vi "Set Button Positions.vi"(4 "Left":i16, 6 "Top":i32, 8 "error in":errorcluster, 10 "label array in":string[](array[string]), 11 "controls[] in":refnum<vi>[](array[refnum])) -> (0 "error out":errorcluster)   [LabVIEW 2018]
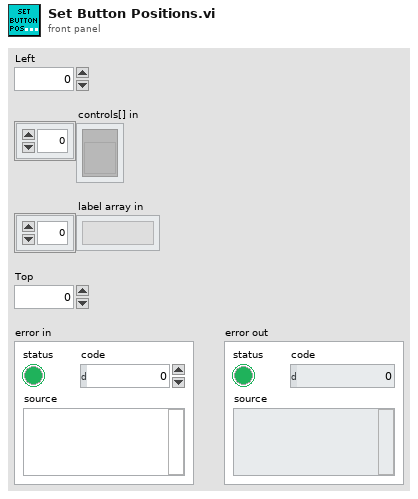
[diagram p1: front panel]
types:
  T1 = typedef "LVRectTypeDef.ctl" = cluster{"Left":i16, "Top":i16, "Right":i16, "Bottom":i16}
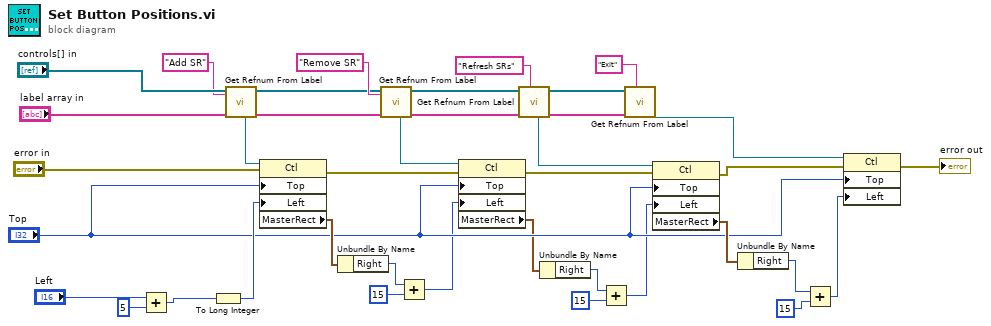
[diagram p0: block diagram]
diagram:
  n1 = Add(x="Left", y=i16 5) -> (x+y=w2:i16)
  n2 = To Long Integer(number=w2) -> (32bit integer=w20:i32)
  n3 = call "Get Refnum From Label.vi"("label"="Add SR" ("element"), "label array in"="label array in", "controls[] in"="controls[] in") -> ("label array out"=w16:string[], "controls[] out"=w17:refnum<vi>[], "refnum out"=w32:refnum<vi>)  [unwired: 6 in]
  n4 = property class="Ctl"(reference=w32, error in="error in", "Top"="Top", "Left"=w20) -> (error out=w13:errorcluster, "MasterRect"=w28:T1)  [unwired: 1 out]
  n5 = Unbundle By Name(w28) -> ("Right"=w29:i16)
  n6 = call "Get Refnum From Label.vi"("label"="Remove SR" ("element"), "label array in"=w16, "controls[] in"=w17) -> ("label array out"=w15:string[], "controls[] out"=w14:refnum<vi>[], "refnum out"=w4:refnum<vi>)  [unwired: 6 in]
  n7 = Add(x=w29, y=i16 15) -> (x+y=w9:i16)
  n8 = property class="Ctl"(reference=w4, error in=w13, "Top"="Top", "Left"=w9) -> (error out=w11:errorcluster, "MasterRect"=w6:T1)  [unwired: 1 out]
  n9 = call "Get Refnum From Label.vi"("label"="Refresh SRs" ("element"), "label array in"=w15, "controls[] in"=w14) -> ("label array out"=w36:string[], "controls[] out"=w37:refnum<vi>[], "refnum out"=w35:refnum<vi>)  [unwired: 6 in]
  n10 = Unbundle By Name(w6) -> ("Right"=w7:i16)
  n11 = Add(x=w7, y=i16 15) -> (x+y=w5:i16)
  n12 = call "Get Refnum From Label.vi"("label"="Exit" ("element"), "label array in"=w36, "controls[] in"=w37) -> ("refnum out"=w34:refnum<vi>)  [unwired: 6 in, 2 out]
  n13 = property class="Ctl"(reference=w35, error in=w11, "Top"="Top", "Left"=w5) -> (error out=w10:errorcluster, "MasterRect"=w23:T1)  [unwired: 1 out]
  n14 = Unbundle By Name(w23) -> ("Right"=w22:i16)
  n15 = Add(x=w22, y=i16 15) -> (x+y=w21:i16)
  n16 = property class="Ctl"(reference=w34, error in=w10, "Top"="Top", "Left"=w21) -> (error out=→"error out":errorcluster)  [unwired: 1 out]
